vi "WILT Update Panel.vi"(8 "error in (no error)":errorcluster, 9 "GUI Aisle 1A (SLAT).":T3[](array[typedef]) {"Night Cycle Count" format="%04d"; "Day Cycle Count" format="%04d"}, 10 "Location Index":i32, 11 "File Locations":T1[](array[typedef])) -> (0 "error out":errorcluster, 2 "Station Data Out":T3 {"Night Cycle Count" format="%04d"; "Day Cycle Count" format="%04d"}, 3 "Button Location":i32)   [LabVIEW 2016]
uses:
  Type Definitions/WILT Dryer.ctl
  Type Definitions/WILT Dryer Details.ctl
  Type Definitions/WILT Agilent Channel Definition.ctl
  Type Definitions/WILT DAQ Data.ctl
  Utility/Save File/File Setup (Public)/Type Definition/Save File DOE File Path Control.ctl
  Utility/Save File/File Setup (Public)/Type Definition/Save File DOE Data Save Filepaths.ctl
  Utility/Save File/File Setup.lvlib
panel:
  # "Day"
  # "Night"
  # "Day"
  # "Night"
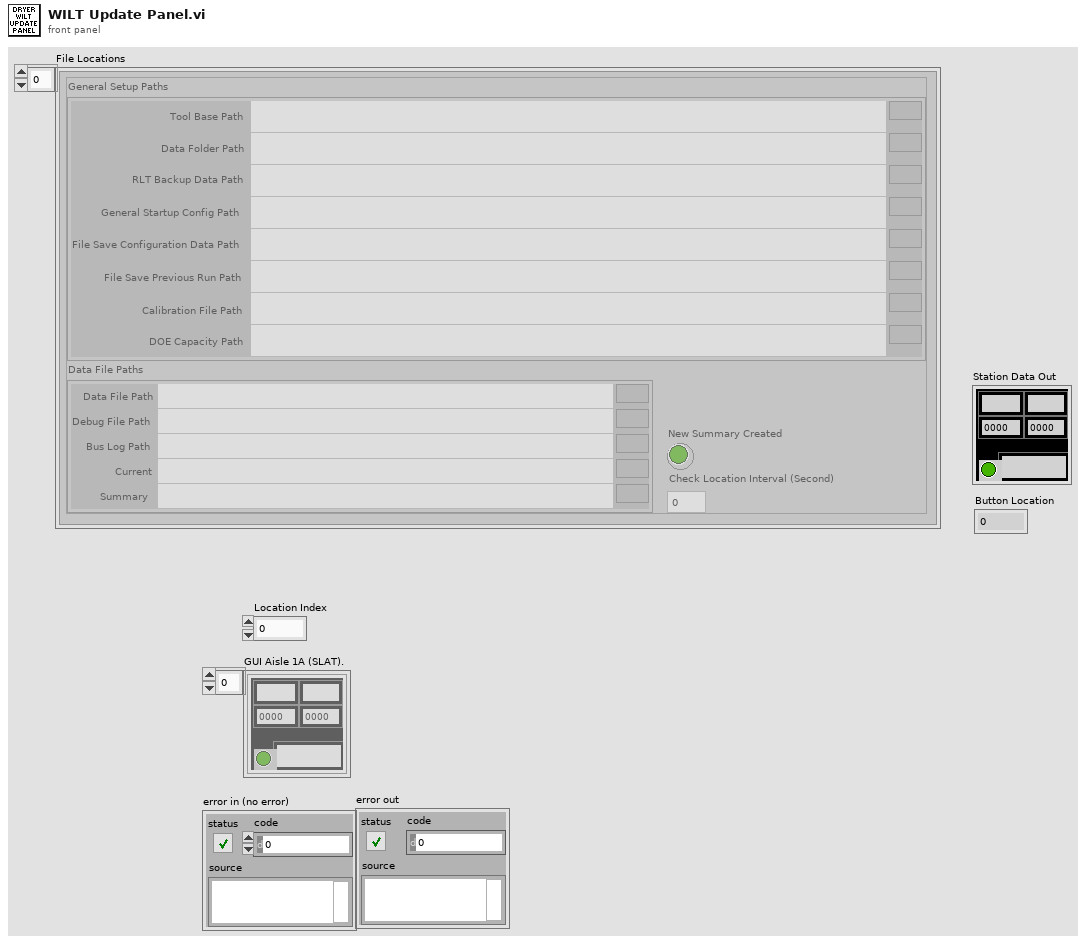
[diagram p1: front panel]
types:
  T1 = typedef "File Setup.lvlib/Save File DOE File Path Control.ctl" = cluster{"General Setup Paths":cluster{"Calibration File Path":path, "DOE Capacity Path":path, "Data Folder Path":path, "RLT Backup Data Path":path, "Tool Base Path":path, "General Startup Config Path":path, "File Save Previous Run Path":path, "File Save Configuration Data Path":path}, "Data File Paths":T2, "New Summary Created":bool, "Check Location Interval (Second)":i32}
  T2 = typedef "File Setup.lvlib/Save File DOE Data Save Filepaths.ctl" = cluster{"Data File Path":path, "Debug File Path":path, "Bus Log Path":path, "Current":path, "Summary":path}
  T3 = typedef "WILT Dryer.ctl" = cluster{"Lab ID":string, "Day Cycle Count":i32, "Station Label":string, "Dryer Details":T4, "Status Color":u32, "Invisible Button":bool, "Night Cycle Count":i32, "Station Index":i32, "Cycle Index":string, "Audit Alert":bool, "Agilent Channel Definition":T5, "DAQ Data":T6}
  T4 = typedef "WILT Dryer Details.ctl" = cluster{"Station":string, "Lab ID":string, "TR Number":string}
  T5 = typedef "WILT Agilent Channel Definition.ctl" = cluster{"Channel":string, "Station":string, "Label":string, "Agilent Station":string, "Data":dbl}
  T6 = typedef "WILT DAQ Data.ctl" = cluster{"L1 Current":dbl, "L2 Current":dbl, "Temperature  Deg F (TC)":dbl, "Volts":dbl, "Volts (208)":dbl, "SW (208)":dbl}
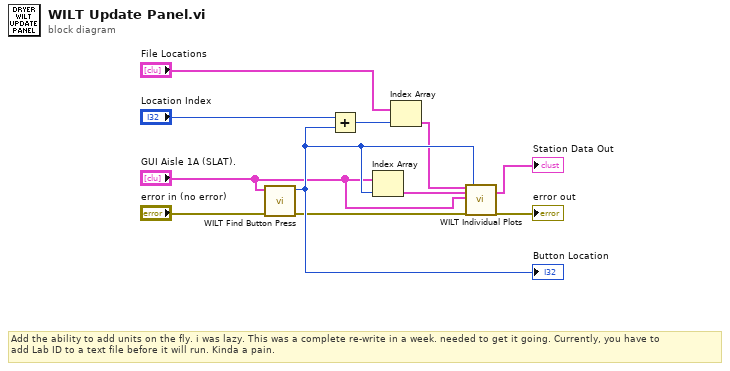
[diagram p0: block diagram]
diagram:
  # "Add the ability to add units on the fly. i was lazy. This was a complete re-write in a week. needed to get it going. Currently, you have to \nadd Lab ID to a text file before it will run. Kinda a pain."
  n1 = call "WILT Find Button Press .vi"("error in (no error)"="error in (no error)", "NewVal"="GUI Aisle 1A (SLAT).") -> ("error out"=w4:errorcluster, "Button Location"=w11:i32)  [unwired: 7 in, 1 out]
  "Button Location" <- w11
  n2 = Add(x="Location Index", y=w11) -> (x+y=w8:i32)
  n3 = Index Array(array="GUI Aisle 1A (SLAT).", index=w11) -> (element=w3:T3)
  n4 = Index Array(array="File Locations", index=w8) -> (element=w2:T1)
  n5 = call "WILT Individual Plots.vi"("File Name"=w2, "Station Data"=w3, "GUI Aisle 1 (SLAT)."="GUI Aisle 1A (SLAT).", "Error In"=w4, "Station Index"=w11) -> ("Station Data Out"=→"Station Data Out":T3, "Error Out"=→"error out":errorcluster)  [unwired: 12 in, 1 out]
